vi "Manually identifying peaks.vi"() -> ()   [LabVIEW 2015]
doc: "Intended use:\n-Displays collected data\n-Attempts a fit to background; separates signal from background\n-Allows user to select a subarray of data with cursors\n-Fits the signal from this subarray to a specified function (in this case, a Lorentzian) and outputs the fit parameters"
uses:
  <vilib>/Utility/file.llb/Read From Spreadsheet File (DBL).vi
panel:
  out "active row":i32
  out "Array":dbl[][](array[numeric])
  out "*(type *) &x":string
  out "Char":i16
  out "Boolean":bool
  out "best fit params":dbl[](array[numeric])
  out "initial params":dbl[](array[numeric])
  out "Subset and Fit":T1(graph)
  out "Data and BG":cluster{"all rows":dbl[], "all rows":dbl[]}[](graph)
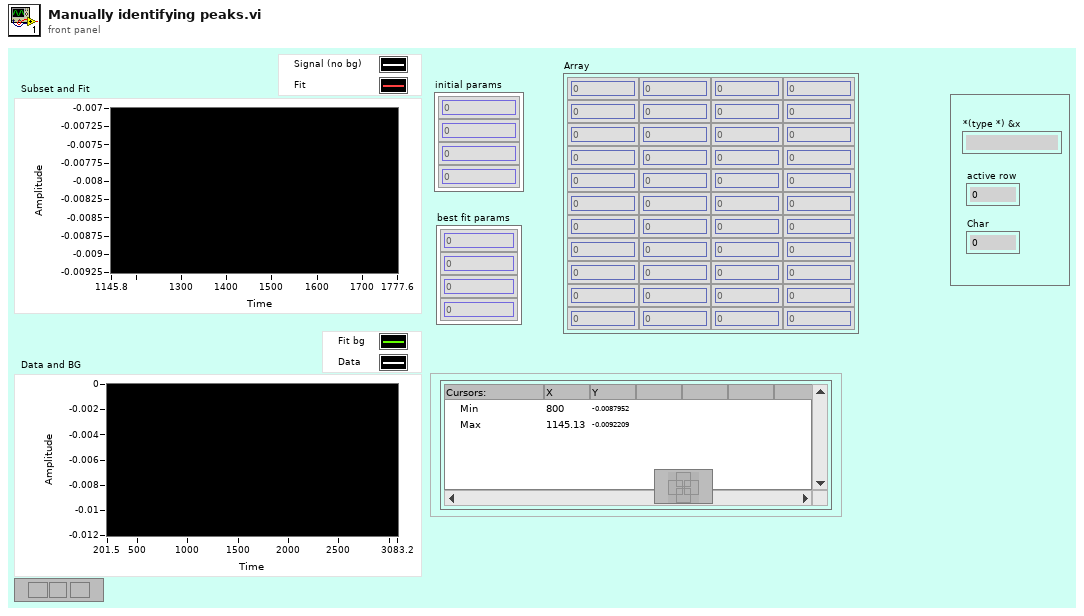
[diagram p1: front panel]
types:
  T1 = cluster{"X subset":dbl[], "best nonlinear fit":dbl[]}[]
  T2 = typedef "eventvkey.ctl" = enum16{"ASCII", "Enter", "Return", "Shift", "Ctrl", "Alt", "Cmd", "Opt", "Caps", "NumLock", "Clear", "Break", "Up", "Down", "Left", "Right", "Insert", "Delete", "Home", "End", "PageUp", "PageDown", "Escape", "Help", "Pause", "ScrollLock", "F1", "F2", "F3", "F4", "F5", "F6", "F7", "F8", "F9", "F10", "F11", "F12", "F13", "F14", "F15", "F16", "F17", "F18", "F19", "F20", "F21", "F22", "F23", "F24", "Play", "VolumeUp", "VolumeDown", "Mute", "Two Byte Char"}
  T3 = typedef "LVPoint32TypeDef.ctl" = cluster{"Horizontal":i32, "Vertical":i32}
  T4 = cluster{"X subset":dbl[], "best nonlinear fit":dbl[]}
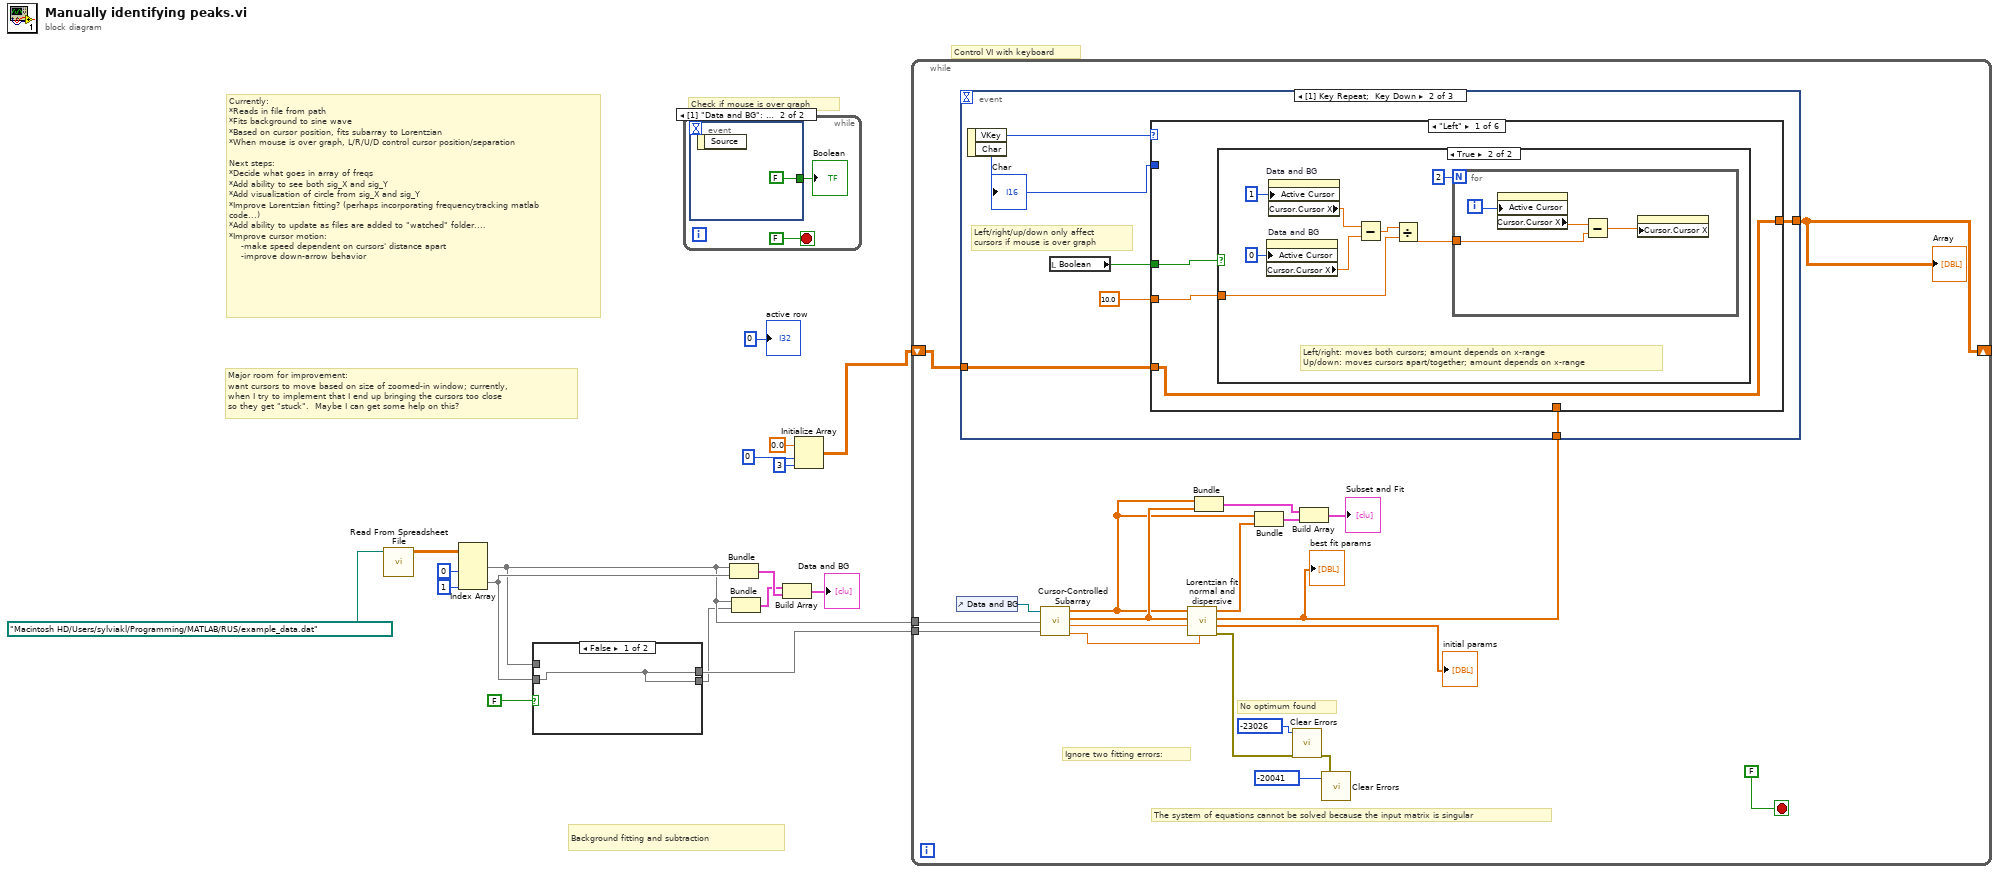
[diagram p0: block diagram]
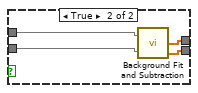
[diagram p2: hidden frame]
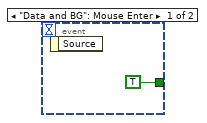
[diagram p3: hidden frame]
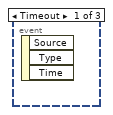
[diagram p4: hidden frame]
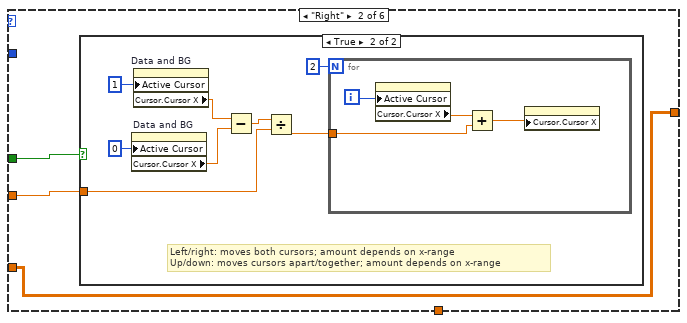
[diagram p6: hidden frame]
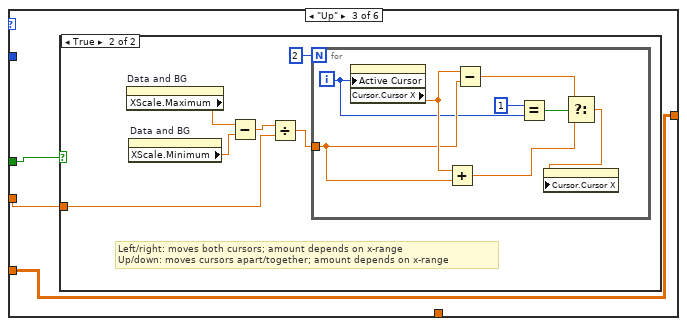
[diagram p8: hidden frame]
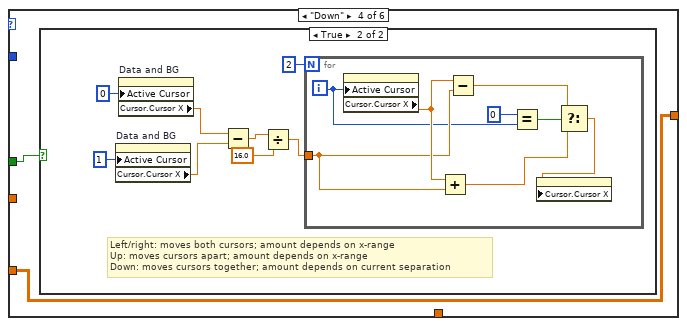
[diagram p10: hidden frame]
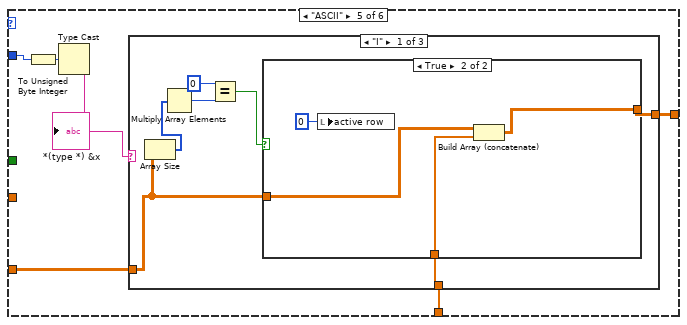
[diagram p12: hidden frame]
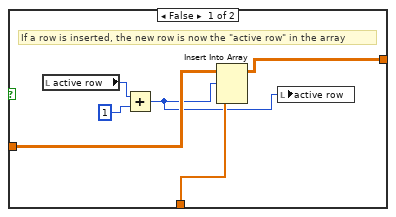
[diagram p13: hidden frame]
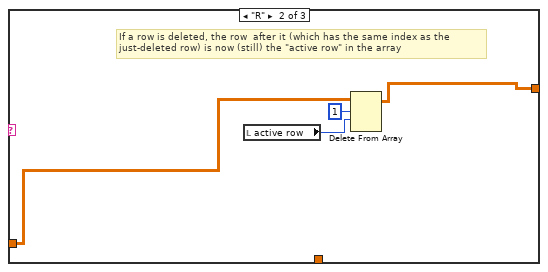
[diagram p14: hidden frame]
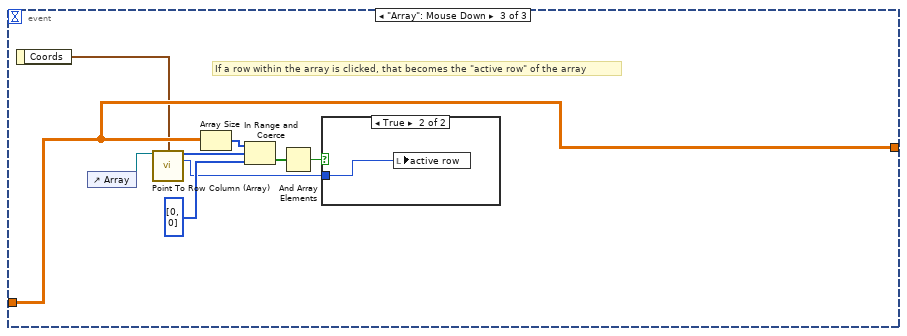
[diagram p17: hidden frame]
diagram:
  # "Background fitting and subtraction"
  # "Currently:\n*Reads in file from path\n*Fits background to sine wave\n*Based on cursor position, fits subarray to Lorentzian\n*When mouse is over graph, L/R/U/D control cursor position/separation\n\nNext steps:\n*Decide what goes in array of freqs\n*Add ability to see both sig_X and sig_Y\n*Add visualization of circle from sig_X and sig_Y\n*Improve Lorentzian fitting? (perhaps incorporating frequencytracking matlab code...)\n*Add ability to update as files are added to \"watched\" folder....\n*Improve cursor motion:\n    -make speed dependent on cursors' distance apart\n    -improve down-arrow behavior"
  # "Check if mouse is over graph"
  # "Major room for improvement:\nwant cursors to move based on size of zoomed-in window; currently,\nwhen I try to implement that I end up bringing the cursors too close\nso they get \"stuck\".  Maybe I can get some help on this?"
  # "Control VI with keyboard"
  n1 = call-poly <vilib>:"Read From Spreadsheet File.vi"("file path (dialog if empty)"=path "/Macintosh HD/Users/sylviakl/Programming/MATLAB/RUS/example_data.dat" ("Path")) -> ("all rows"=w15:dbl[][])  [unwired: 6 in, 4 out]
  n2 = Index Array(array=w15, index (col) #1=0 ("disabled index (col)"), index (col) #2=1 ("index (col)")) -> (element #1=w13:dbl[], element #2=w14:dbl[])  [unwired: 2 in]
  n3 = case shown="False" FALSE {
    tunnel: w14 -> [w18 w22]
    tunnel: w13 -> [_ w21]
    tunnel: [w18 w20] -> w11
    tunnel: [w18 w19] -> w10
    frame False {
    }
    frame True {
      n4 = call "Background Fit and Subtraction.vi"("X"=w21, "Y"=w22) -> ("signal"=w20:dbl[], "background"=w19:dbl[])  [unwired: 1 out]
    }
  }
  n5 = while {
    stop <- FALSE stop-if-true
    n6 = event shown="[1] \"Data and BG\": Mouse Leave" {
      selector: _ -> [_ _]
      dyn-events: _ -> [_ _]
      timeout: _ -> [_ _]
      tunnel: [TRUE FALSE] -> w23
      event "Data and BG": Mouse Enter {
        n7 = event-data() -> ()  [unwired: 1 in, 1 out]
      }
      event "Data and BG": Mouse Leave {
        n8 = event-data() -> ()  [unwired: 1 in, 1 out]
      }
    }
    "Boolean" <- w23
  }
  n9 = Bundle("all rows"=w13, "all rows"=w14) -> (w9:cluster{"all rows":dbl[], "all rows":dbl[]})  [unwired: 1 in]
  n10 = Bundle("all rows"=w13, "background"=w10) -> (w8:cluster{"all rows":dbl[], "background":dbl[]})  [unwired: 1 in]
  n11 = Build Array(w8, w9) -> (→"Data and BG":cluster{"all rows":dbl[], "all rows":dbl[]}[])
  n12 = Initialize Array(0.0 ("element"), 0 ("dimension size"), 3 ("dimension size")) -> (w3:dbl[][])
  n13 = while {
    tunnel: w13 -> [w41]
    tunnel: w11 -> [w40]
    shift-right: [w35] -> _
    shift-left: w3 -> [w34]
    stop <- FALSE stop-if-true
    # "The system of equations cannot be solved because the input matrix is singular"
    # "Ignore two fitting errors:"
    # "No optimum found"
    n14 = control-ref of="Data and BG"() -> (w39:refnum<vi>)
    n15 = call "Cursor-Controlled Subarray.vi"("cursor graph"=w39, "X"=w41, "Y"=w40) -> ("X subset"=w32:dbl[], "Y subset"=w38:dbl[], "cursor avg"=w36:dbl, "cursor diff"=w37:dbl)
    n16 = call "Lorentzian fit normal and dispersive.vi"("cursor diff"=w37, "cursor avg"=w36, "Y subset"=w38, "X subset"=w32) -> ("error out"=w31:errorcluster, "Initial params"=→"initial params":dbl[], "best fit parameters"=w33:dbl[], "best nonlinear fit"=w42:dbl[])  [unwired: 4 in]
    "best fit params" <- w33
    n17 = event shown="[1] Key Repeat;  Key Down" {
      selector: _ -> [_ _ _]
      dyn-events: _ -> [_ _ _]
      timeout: _ -> [_ _ _]
      tunnel: w34 -> [_ w49 w150]
      tunnel: [_ w48 w150] -> w35
      tunnel: w33 -> [_ w47 _]
      event Timeout {
        n18 = event-data() -> ()  [unwired: 1 in, 3 out]
      }
      event Key Repeat; Key Down {
        # "Left/right/up/down only affect\ncursors if mouse is over graph"
        n19 = event-data() -> ("VKey"=w53:T2, "Char"=w52:i16)  [unwired: 1 in]
        "Char" <- w52
        n20 = local read "Boolean"() -> (w50:bool)
        n21 = case shown="\"Left\"" w53 {
          tunnel: w52 -> [_ _ _ _ w124 _]
          tunnel: 10.0 ("y") -> [w56 w71 w86 _ _ _]
          tunnel: w50 -> [w55 w70 w85 w102 _ _]
          tunnel: w49 -> [w54 w69 w84 w101 w121 w147]
          tunnel: [w54 w69 w84 w101 w120 w147] -> w48
          tunnel: w47 -> [_ _ _ _ w119 _]
          frame "Left" {
            n22 = case shown="True" w55 {
              tunnel: w56 -> [_ w61]
              frame False {
              }
              frame True {
                # "Left/right: moves both cursors; amount depends on x-range\nUp/down: moves cursors apart/together; amount depends on x-range"
                n23 = property on="Data and BG" class="XYGraph (strict)"("Active Cursor"=u32 0) -> ("Cursor.Cursor X"=w60:dbl)  [unwired: 2 in, 2 out]
                n24 = property on="Data and BG" class="XYGraph (strict)"("Active Cursor"=u32 1) -> ("Cursor.Cursor X"=w59:dbl)  [unwired: 2 in, 2 out]
                n25 = Subtract(x=w59, y=w60) -> (x-y=w63:dbl)
                n26 = Divide(x=w63, y=w61) -> (x/y=w62:dbl)
                n27 = for {
                  N: 2 -> [_]
                  tunnel: w62 -> [w65]
                  i -> [w66]
                  n28 = property on="Data and BG" class="XYGraph (strict)"("Active Cursor"=w66) -> ("Cursor.Cursor X"=w67:dbl)  [unwired: 2 in, 2 out]
                  n29 = Subtract(x=w67, y=w65) -> (x-y=w68:dbl)
                  n30 = property on="Data and BG" class="XYGraph (strict)"("Cursor.Cursor X"=w68) -> ()  [unwired: 2 in, 2 out]
                }
              }
            }
          }
          frame "Right" {
            n31 = case shown="True" w70 {
              tunnel: w71 -> [_ w76]
              frame False {
              }
              frame True {
                # "Left/right: moves both cursors; amount depends on x-range\nUp/down: moves cursors apart/together; amount depends on x-range"
                n32 = property on="Data and BG" class="XYGraph (strict)"("Active Cursor"=u32 0) -> ("Cursor.Cursor X"=w75:dbl)  [unwired: 2 in, 2 out]
                n33 = property on="Data and BG" class="XYGraph (strict)"("Active Cursor"=u32 1) -> ("Cursor.Cursor X"=w74:dbl)  [unwired: 2 in, 2 out]
                n34 = Subtract(x=w74, y=w75) -> (x-y=w78:dbl)
                n35 = Divide(x=w78, y=w76) -> (x/y=w77:dbl)
                n36 = for {
                  N: 2 -> [_]
                  tunnel: w77 -> [w80]
                  i -> [w81]
                  n37 = property on="Data and BG" class="XYGraph (strict)"("Active Cursor"=w81) -> ("Cursor.Cursor X"=w82:dbl)  [unwired: 2 in, 2 out]
                  n38 = Add(x=w82, y=w80) -> (x+y=w83:dbl)
                  n39 = property on="Data and BG" class="XYGraph (strict)"("Cursor.Cursor X"=w83) -> ()  [unwired: 2 in, 2 out]
                }
              }
            }
          }
          frame "Up" {
            n40 = case shown="True" w85 {
              tunnel: w86 -> [_ w87]
              frame False {
              }
              frame True {
                # "Left/right: moves both cursors; amount depends on x-range\nUp/down: moves cursors apart/together; amount depends on x-range"
                n41 = property on="Data and BG" class="XYGraph (strict)"() -> ("XScale.Maximum"=w90:dbl)  [unwired: 2 in, 2 out]
                n42 = property on="Data and BG" class="XYGraph (strict)"() -> ("XScale.Minimum"=w89:dbl)  [unwired: 2 in, 2 out]
                n43 = Subtract(x=w90, y=w89) -> (x-y=w91:dbl)
                n44 = Divide(x=w91, y=w87) -> (x/y=w88:dbl)
                n45 = for {
                  N: 2 -> [_]
                  tunnel: w88 -> [w99]
                  i -> [w94]
                  n46 = property on="Data and BG" class="XYGraph (strict)"("Active Cursor"=w94) -> ("Cursor.Cursor X"=w100:dbl)  [unwired: 2 in, 2 out]
                  n47 = Add(x=w100, y=w99) -> (x+y=w97:dbl)
                  n48 = Subtract(x=w100, y=w99) -> (x-y=w98:dbl)
                  n49 = Equal?(x=1, y=w94) -> (x = y?=w95:bool)
                  n50 = Select(t=w98, s=w95, f=w97) -> (s? t:f=w96:dbl)
                  n51 = property on="Data and BG" class="XYGraph (strict)"("Cursor.Cursor X"=w96) -> ()  [unwired: 2 in, 2 out]
                }
              }
            }
          }
          frame "Down" {
            n52 = case shown="True" w102 {
              frame False {
              }
              frame True {
                # "Left/right: moves both cursors; amount depends on x-range\nUp: moves cursors apart; amount depends on x-range\nDown: moves cursors together; amount depends on current separation"
                n53 = property on="Data and BG" class="XYGraph (strict)"("Active Cursor"=u32 1) -> ("Cursor.Cursor X"=w106:dbl)  [unwired: 2 in, 2 out]
                n54 = property on="Data and BG" class="XYGraph (strict)"("Active Cursor"=u32 0) -> ("Cursor.Cursor X"=w105:dbl)  [unwired: 2 in, 2 out]
                n55 = Subtract(x=w105, y=w106) -> (x-y=w109:dbl)
                n56 = Divide(x=w109, y=16.0) -> (x/y=w108:dbl)
                n57 = for {
                  N: 2 -> [_]
                  tunnel: w108 -> [w117]
                  i -> [w112]
                  n58 = property on="Data and BG" class="XYGraph (strict)"("Active Cursor"=w112) -> ("Cursor.Cursor X"=w118:dbl)  [unwired: 2 in, 2 out]
                  n59 = Add(x=w118, y=w117) -> (x+y=w115:dbl)
                  n60 = Subtract(x=w118, y=w117) -> (x-y=w116:dbl)
                  n61 = Equal?(x=0, y=w112) -> (x = y?=w113:bool)
                  n62 = Select(t=w116, s=w113, f=w115) -> (s? t:f=w114:dbl)
                  n63 = property on="Data and BG" class="XYGraph (strict)"("Cursor.Cursor X"=w114) -> ()  [unwired: 2 in, 2 out]
                }
              }
            }
          }
          frame "ASCII" {
            n64 = To Unsigned Byte Integer(number=w124) -> (unsigned 8bit integer=w122:u8)
            n65 = Type Cast(x=w122) -> (*(type *) &x=w123:string)  [unwired: 1 in]
            "*(type *) &x" <- w123
            n66 = case shown="\"I\"" w123 {
              tunnel: w121 -> [w129 w144 w146]
              tunnel: [w130 w145 w146] -> w120
              tunnel: w119 -> [w131 _ _]
              frame "I" {
                n67 = Array Size(array=w129) -> (size(s)=w127:i32[])
                n68 = Multiply Array Elements(1:w127) -> (0:w128:i32)
                n69 = Equal?(x=0, y=w128) -> (x = y?=w125:bool)
                n70 = case shown="True" w125 {
                  tunnel: w129 -> [w137 w139]
                  tunnel: w131 -> [w134 w140]
                  tunnel: [w133 w138] -> w130
                  frame False {
                    # "If a row is inserted, the new row is now the \"active row\" in the array"
                    n71 = local read "active row"() -> (w135:i32)
                    n72 = Add(x=w135, y=1) -> (x+y=w132:i32)
                    n73 = Insert Into Array(array=w137, index (row)=w132, new element=w134) -> (w133:dbl[][])  [unwired: 1 in]
                    n74 = local write "active row"(w132) -> ()
                  }
                  frame True {
                    n75 = local write "active row"(0 ("active row")) -> ()
                    n76 = Build Array (concatenate)(w139, w140) -> (w138:dbl[][])
                  }
                }
              }
              frame "R" {
                # "If a row is deleted, the row  after it (which has the same index as the just-deleted row) is now (still) the \"active row\" in the array"
                n77 = local read "active row"() -> (w142:i32)
                n78 = Delete From Array(array=w144, length=1, index (row)=w142) -> (array with subset deleted=w145:dbl[][])  [unwired: 1 in, 1 out]
              }
              frame Default {
              }
            }
          }
          frame Default {
          }
        }
      }
      event "Array": Mouse Down {
        # "If a row within the array is clicked, that becomes the \"active row\" of the array"
        n79 = event-data() -> ("Coords"=w149:T3)  [unwired: 1 in]
        n80 = control-ref of="Array"() -> (w148:refnum<vi>)
        n81 = call "Point To Row Column (Array).vi"("reference"=w148, "Coords of Click"=w149) -> ("Clicked Index"=w154:i32[], "Clicked Row"=w151:i32)  [unwired: 8 in, 4 out]
        n82 = Array Size(array=w150) -> (size(s)=w153:i32[])
        n83 = In Range and Coerce(upper limit=w153, x=w154, lower limit=i32[] [0, 0]) -> (In Range?=w155:bool[])  [unwired: 1 out]
        n84 = And Array Elements(Boolean array=w155) -> (logical AND=w152:bool)
        n85 = case shown="True" w152 {
          tunnel: w151 -> [_ w157]
          frame False {
          }
          frame True {
            n86 = local write "active row"(w157) -> ()
          }
        }
      }
    }
    "Array" <- w35
    n87 = Bundle("X subset"=w32, "Y subset"=w38) -> (w44:cluster{"X subset":dbl[], " Y subset":dbl[]})  [unwired: 1 in]
    n88 = Bundle("X subset"=w32, "best nonlinear fit"=w42) -> (w43:T4)  [unwired: 1 in]
    n89 = call <vilib>:"Clear Errors.vi"("error in (no error)"=w31, "specific error code to clear (0: all)"=-23026 ("[exception code]")) -> ("error out"=w30:errorcluster)  [unwired: 4 in, 1 out]
    n90 = Build Array(w44, w43) -> (→"Subset and Fit":T1)
    n91 = call <vilib>:"Clear Errors.vi"("error in (no error)"=w30, "specific error code to clear (0: all)"=-20041 ("[exception code]")) -> ()  [unwired: 4 in, 2 out]
  }
  "active row" <- 0 ("dimension size")
